vi "systemExec.vi"() -> ()   [LabVIEW 2014]
panel:
  out "Python Invocation \nError":errorcluster
  out "File Deletion \nError":errorcluster
  in  "Command line arguments":string
  out "Python Error Messages":string
  out "Python Output":string
  in  "Python Code":string
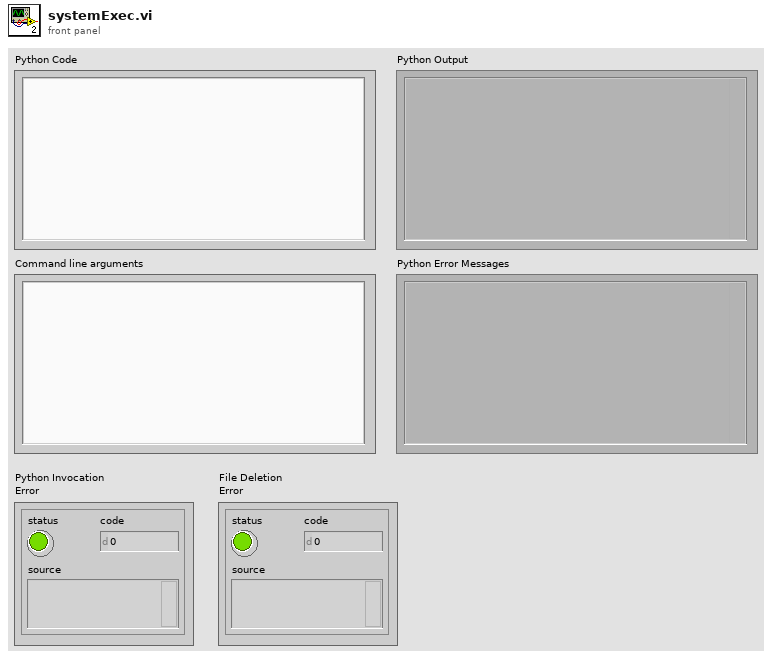
[diagram p1: front panel]
types:
  T1 = enum16{"open", "replace", "create", "open or create", "replace or create", "replace or create with confirmation"}
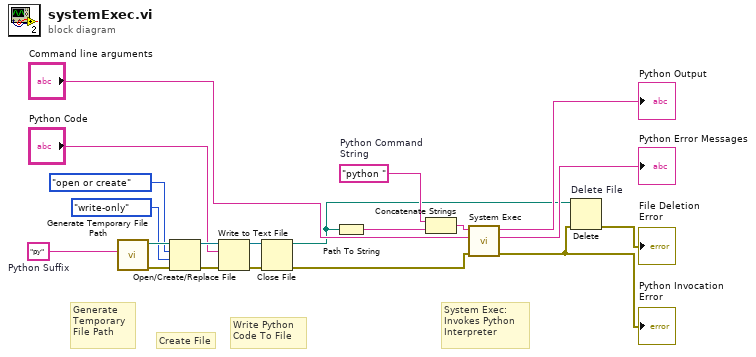
[diagram p0: block diagram]
diagram:
  w13 = "python "  # Python Command  String
  w20 = "py"  # Python Suffix
  # "System Exec:\nInvokes Python \nInterpreter"
  # "Write Python \nCode To File"
  # "Create File"
  # "Generate \nTemporary \nFile Path"
  n1 = call <vilib>:"Generate Temporary File Path.vi"("Temporary File Extension (tmp)"=w20) -> ("error out"=w18:errorcluster, "Unique Temporary File Path"=w19:path)  [unwired: 9 in]
  n2 = Open/Create/Replace File(file path (use dialog)=w19, error in=w18, operation (0:open)=T1."open or create", access (0:read/write)=enum16{"read/write", "read-only", "write-only"}."write-only") -> (refnum out=w16:refnum<file>, error out=w14:errorcluster)  [unwired: 2 in, 1 out]
  n3 = Write to Text File(file (use dialog)=w16, text="Python Code", error in=w14) -> (refnum out=w10:refnum<file>, error out=w9:errorcluster)  [unwired: 1 in, 1 out]
  n4 = Close File(refnum=w10, error in=w9) -> (path=w4:path, error out=w8:errorcluster)
  n5 = Path To String(path=w4) -> (string=w12:string)
  n6 = Concatenate Strings(w13, w12) -> (w11:string)
  n7 = call <vilib>:"System Exec.vi"("error in (no error)"=w8, "standard input"="Command line arguments", "command line"=w11) -> ("error out"=w2:errorcluster, "standard error"=→"Python Error Messages":string, "standard output"=→"Python Output":string)  [unwired: 5 in, 1 out]
  "Python Invocation \nError" <- w2
  n8 = Delete "Delete File"(path (use dialog)=w4, error in=w2) -> (error out=→"File Deletion \nError":errorcluster)  [unwired: 3 in, 2 out]
